vi "Encode Image.vi"   [LabVIEW 2020, in "image.lvlib" / "Image to File-Buffer Encoder.lvclass"]
uses:
  Image to File-Buffer Encoder.lvclass
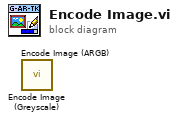
[diagram p0: block diagram]
diagram:
  n1 = call "Encode Image (Greyscale).vi"() -> ()  [unwired: 9 in, 3 out]
  n2 = call "Encode Image (ARGB).vi"() -> ()  [unwired: 9 in, 3 out]
